vi "rapid_mode_test.vi"() -> ()   [LabVIEW 2013]
uses:
  Controls/PicoScope/pico_control_panel.ctl
  Controls/PicoScope/pico_channel_settings.ctl
  Controls/PicoScope/pico_trigger.ctl
  Controls/PicoScope/pico_init_settings.ctl
panel:
  out "Pico A":T1(graph)
  out "Pico B":T1(graph)
  in  "PicoScope Acquisition Settings":T2={"Channel A Settings"={"Enabled"=TRUE, "Coupling"=1, "Range"=6, "Analogue Offset"=0.0}, "Channel B Settings"={"Enabled"=TRUE, "Coupling"=1, "Range"=6, "Analogue Offset"=0.0}, "Trigger Options"={"Trigger Enabled"=FALSE, "Trigger Source"=enum."Channel A", "Trigger Threshold (-5 to 5 V)"=0.0, "Trigger Slope"=2, "Trigger Delay (ms)"=0.0, "Auto Trigger Time (ms)"=1000}, "Pico Scope Inititalization Settings"={"USB Power"=FALSE, "Use Serial Number"=FALSE, "Resolution"=0, "Serial Number"="", "Handle"=0}, "Use PicoScope?"=FALSE, "Acquisition Settings"={"Pre Trigger Time (s)"=512.0, "Post Trigger Time (s)"=512.0, "Resolution (s)"=34.36, "Four Channel Device"=FALSE, "Number of Captures"=1.0}} {"Acquisition Settings"."Number of Captures" min=1.0 step=1.0; "Acquisition Settings"."Resolution (s)" min=8e-09 max=34.36 step=8e-09 format="%#_6p"; "Acquisition Settings"."Post Trigger Time (s)" min=0.0 format="%#_6p"; "Acquisition Settings"."Pre Trigger Time (s)" min=0.0 format="%#_6p"; "Pico Scope Inititalization Settings"."Resolution" items=["8-bit", "12-bit", "14-bit", "15-bit (max. 2 ch.)", "16-bit (max. 1 ch.)"]; "Trigger Options"."Trigger Slope" items=["Rising"=2, "Falling"=3]; "Channel B Settings"."Range" items=["10 mV", "20 mV", "50 mV", "100 mV", "200 mV", "500 mV", "1 V", "2 V", "5 V", "10 V", "20 V", "50 V ", "100 V"]; "Channel B Settings"."Coupling" items=["AC", "DC"]; "Channel A Settings"."Range" items=["10 mV", "20 mV", "50 mV", "100 mV", "200 mV", "500 mV", "1 V", "2 V", "5 V", "10 V", "20 V", "50 V ", "100 V"]; "Channel A Settings"."Coupling" items=["AC", "DC"]}
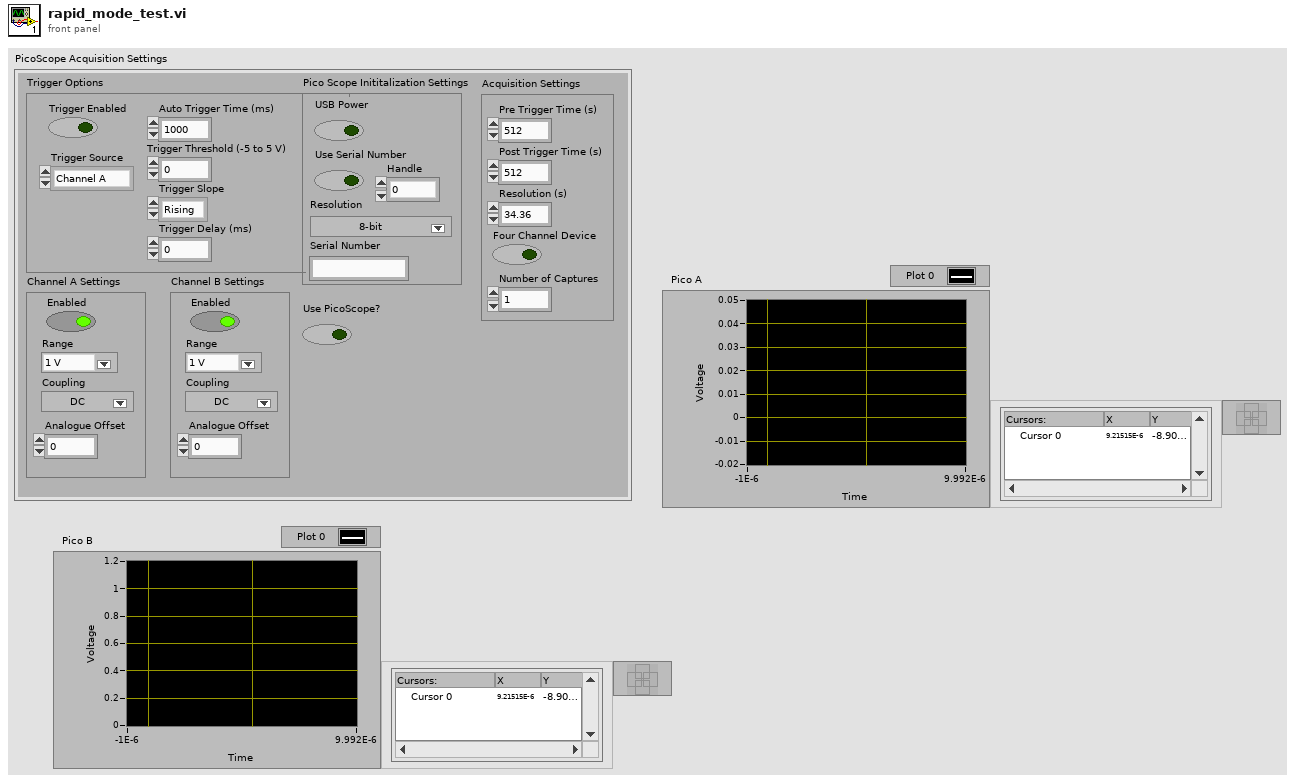
[diagram p1: front panel]
types:
  T1 = cluster{"Channel A Out":dbl[], "Channel A Out":dbl[]}[]
  T2 = typedef "pico_control_panel.ctl" = cluster{"Channel A Settings":T3, "Channel B Settings":T3, "Trigger Options":T4, "Pico Scope Inititalization Settings":T5, "Use PicoScope?":bool, "Acquisition Settings":cluster{"Pre Trigger Time (s)":dbl, "Post Trigger Time (s)":dbl, "Resolution (s)":dbl, "Four Channel Device":bool, "Number of Captures":dbl}}
  T3 = typedef "pico_channel_settings.ctl" = cluster{"Enabled":bool, "Coupling":i16, "Range":u16, "Analogue Offset":sgl}
  T4 = typedef "pico_trigger.ctl" = cluster{"Trigger Enabled":bool, "Trigger Source":enum16{"Channel A", "Channel B", "Channel C", "Channel D", "Ext."}, "Trigger Threshold (-5 to 5 V)":dbl, "Trigger Slope":u16, "Trigger Delay (ms)":dbl, "Auto Trigger Time (ms)":i16}
  T5 = typedef "pico_init_settings.ctl" = cluster{"USB Power":bool, "Use Serial Number":bool, "Resolution":i32, "Serial Number":string, "Handle":i16}
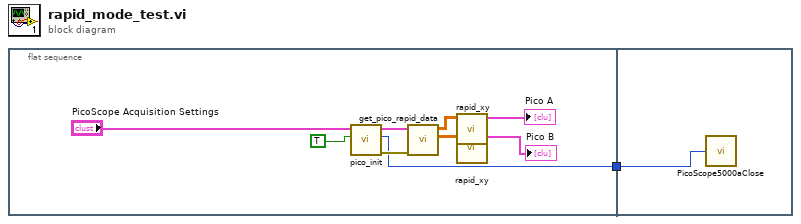
[diagram p0: block diagram]
diagram:
  n1 = flat-sequence {
    tunnel: [w2] -> w1
    tunnel: w1 -> [w11]
    frame #0 {
      n2 = call "pico_init.vi"("Initialize PicoScope?"=TRUE ("Boolean"), "PicoScope Acquisition Settings"="PicoScope Acquisition Settings") -> ("error out"=w3:errorcluster, "Handle Out"=w2:i16, "PicoScope Acquisition Settings 2"=w4:T2)  [unwired: 5 in, 1 out]
      n3 = call "get_pico_rapid_data.vi"("error in"=w3, "PicoScope Acquisition Settings"=w4) -> ("Channel B Out"=w9:dbl[][][], "Channel A Out"=w10:dbl[][][])  [unwired: 7 in, 1 out]
      n4 = call "rapid_xy.vi"("Channel A Out"=w10) -> ("xy array"=→"Pico A":T1)  [unwired: 10 in]
      n5 = call "rapid_xy.vi"("Channel A Out"=w9) -> ("xy array"=→"Pico B":T1)  [unwired: 10 in]
    }
    frame #1 {
      n6 = call <userlib>:"PicoScope5000aClose.vi"("handle"=w11) -> ()
    }
  }
